vi "Set Shooter RPM.vi"(6 "Key Shot":bool, 8 "Open Loop":bool, 9 "Increment":bool, 10 "Decrement":bool, 11 "Shooter Enabled":bool) -> ()   [LabVIEW 2011]
uses:
  System Set Points and States.vi
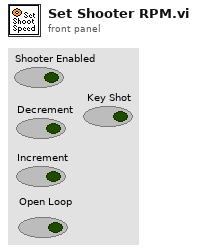
[diagram p1: front panel]
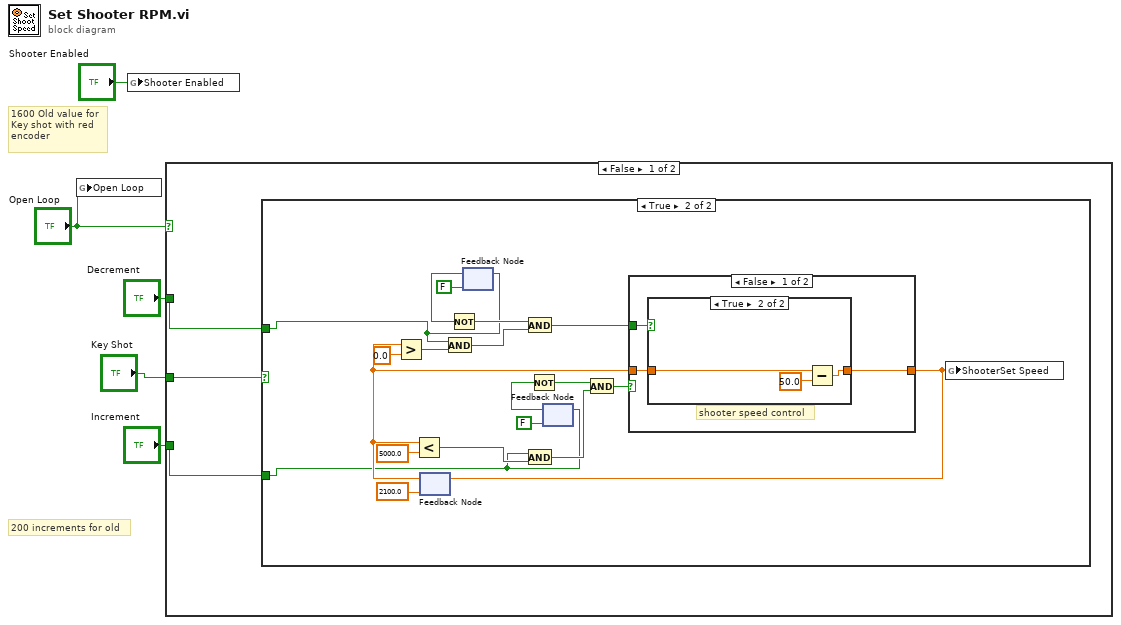
[diagram p0: block diagram]
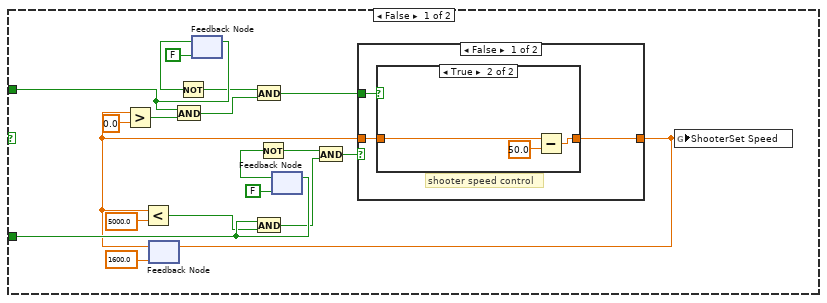
[diagram p2: hidden frame]
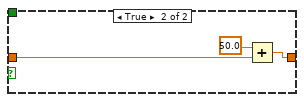
[diagram p4: hidden frame]
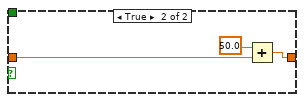
[diagram p6: hidden frame]
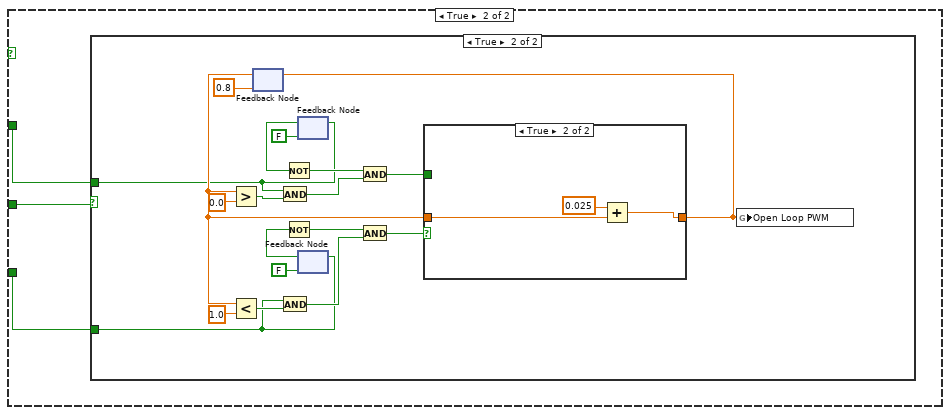
[diagram p7: hidden frame]
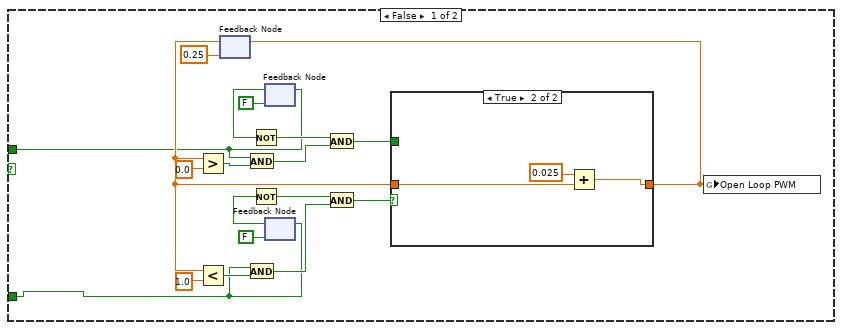
[diagram p8: hidden frame]
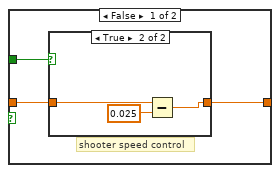
[diagram p9: hidden frame]
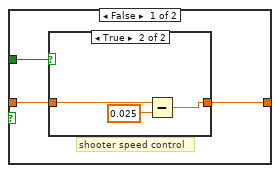
[diagram p11: hidden frame]
diagram:
  # "200 increments for old"
  # "1600 Old value for\nKey shot with red\nencoder"
  n1 = global write "System Set Points and States.vi" "Open Loop"("Open Loop") -> ()
  n2 = global write "System Set Points and States.vi" "Shooter Enabled"("Shooter Enabled") -> ()
  n3 = case shown="False" "Open Loop" {
    tunnel: "Decrement" -> [w8 w69]
    tunnel: "Increment" -> [w7 w68]
    tunnel: "Key Shot" -> [w6 w67]
    frame False {
      n4 = case shown="True" w6 {
        tunnel: w8 -> [w27 w38]
        tunnel: w7 -> [w26 w39]
        frame False {
          n5 = feedback #1(1600.0) -> (w11:dbl)
          n6 = Greater?(x=w11, y=0.0) -> (0:w9:bool)
          n7 = Less?(x=w11, y=5000.0) -> (x < y?=w12:bool)
          n8 = And(x=w27, y=w9) -> (x .and. y?=w18:bool)
          n9 = feedback #2(FALSE) -> (w22:bool)
          n10 = Not(x=w22) -> (.not. x?=w23:bool)
          n11 = feedback-in #2(w27) -> ()
          n12 = And(x=w23, y=w18) -> (x .and. y?=w19:bool)
          n13 = And(x=w26, y=w12) -> (x .and. y?=w15:bool)
          n14 = feedback #3(FALSE) -> (w20:bool)
          n15 = Not(x=w20) -> (.not. x?=w21:bool)
          n16 = feedback-in #3(w26) -> ()
          n17 = And(x=w21, y=w15) -> (x .and. y?=w16:bool)
          n18 = case shown="False" w16 {
            tunnel: w19 -> [w30 _]
            tunnel: w11 -> [w29 w37]
            tunnel: [w28 w35] -> w25
            frame False {
              # "shooter speed control"
              n19 = case shown="True" w30 {
                tunnel: w29 -> [w31 w34]
                tunnel: [w31 w32] -> w28
                frame False {
                }
                frame True {
                  n20 = Subtract(x=w34, y=50.0) -> (x-y=w32:dbl)
                }
              }
            }
            frame True {
              n21 = Add(x=50.0, y=w37) -> (x+y=w35:dbl)
            }
          }
          n22 = feedback-in #1(w25) -> ()
          n23 = global write "System Set Points and States.vi" "ShooterSet Speed"(w25) -> ()
        }
        frame True {
          n24 = feedback #4(2100.0) -> (w42:dbl)
          n25 = Greater?(x=w42, y=0.0) -> (0:w40:bool)
          n26 = Less?(x=w42, y=5000.0) -> (x < y?=w43:bool)
          n27 = And(x=w38, y=w40) -> (x .and. y?=w49:bool)
          n28 = feedback #5(FALSE) -> (w53:bool)
          n29 = Not(x=w53) -> (.not. x?=w54:bool)
          n30 = feedback-in #5(w38) -> ()
          n31 = And(x=w54, y=w49) -> (x .and. y?=w50:bool)
          n32 = And(x=w39, y=w43) -> (x .and. y?=w46:bool)
          n33 = feedback #6(FALSE) -> (w51:bool)
          n34 = Not(x=w51) -> (.not. x?=w52:bool)
          n35 = feedback-in #6(w39) -> ()
          n36 = And(x=w52, y=w46) -> (x .and. y?=w47:bool)
          n37 = case shown="False" w47 {
            tunnel: w50 -> [w59 _]
            tunnel: w42 -> [w58 w66]
            tunnel: [w57 w64] -> w56
            frame False {
              # "shooter speed control"
              n38 = case shown="True" w59 {
                tunnel: w58 -> [w60 w63]
                tunnel: [w60 w61] -> w57
                frame False {
                }
                frame True {
                  n39 = Subtract(x=w63, y=50.0) -> (x-y=w61:dbl)
                }
              }
            }
            frame True {
              n40 = Add(x=50.0, y=w66) -> (x+y=w64:dbl)
            }
          }
          n41 = feedback-in #4(w56) -> ()
          n42 = global write "System Set Points and States.vi" "ShooterSet Speed"(w56) -> ()
        }
      }
    }
    frame True {
      n43 = case shown="True" w67 {
        tunnel: w69 -> [w71 w101]
        tunnel: w68 -> [w70 w100]
        frame False {
          n44 = feedback #7(0.25) -> (w75:dbl)
          n45 = Greater?(x=w75, y=0.0) -> (0:w88:bool)
          n46 = Less?(x=w75, y=1.0) -> (x < y?=w86:bool)
          n47 = And(x=w71, y=w88) -> (x .and. y?=w81:bool)
          n48 = And(x=w70, y=w86) -> (x .and. y?=w83:bool)
          n49 = feedback #8(FALSE) -> (w78:bool)
          n50 = Not(x=w78) -> (.not. x?=w77:bool)
          n51 = feedback-in #8(w71) -> ()
          n52 = feedback #9(FALSE) -> (w80:bool)
          n53 = Not(x=w80) -> (.not. x?=w79:bool)
          n54 = feedback-in #9(w70) -> ()
          n55 = And(x=w77, y=w81) -> (x .and. y?=w74:bool)
          n56 = And(x=w79, y=w83) -> (x .and. y?=w73:bool)
          n57 = case shown="True" w73 {
            tunnel: w74 -> [w91 _]
            tunnel: w75 -> [w90 w98]
            tunnel: [w89 w96] -> w72
            frame False {
              # "shooter speed control"
              n58 = case shown="True" w91 {
                tunnel: w90 -> [w92 w95]
                tunnel: [w92 w93] -> w89
                frame False {
                }
                frame True {
                  n59 = Subtract(x=w95, y=0.025) -> (x-y=w93:dbl)
                }
              }
            }
            frame True {
              n60 = Add(x=0.025, y=w98) -> (x+y=w96:dbl)
            }
          }
          n61 = feedback-in #7(w72) -> ()
          n62 = global write "System Set Points and States.vi" "Open Loop PWM"(w72) -> ()
        }
        frame True {
          n63 = feedback #10(0.8) -> (w104:dbl)
          n64 = Greater?(x=w104, y=0.0) -> (0:w117:bool)
          n65 = Less?(x=w104, y=1.0) -> (x < y?=w115:bool)
          n66 = And(x=w101, y=w117) -> (x .and. y?=w110:bool)
          n67 = And(x=w100, y=w115) -> (x .and. y?=w112:bool)
          n68 = feedback #11(FALSE) -> (w107:bool)
          n69 = Not(x=w107) -> (.not. x?=w106:bool)
          n70 = feedback-in #11(w101) -> ()
          n71 = feedback #12(FALSE) -> (w109:bool)
          n72 = Not(x=w109) -> (.not. x?=w108:bool)
          n73 = feedback-in #12(w100) -> ()
          n74 = And(x=w106, y=w110) -> (x .and. y?=w103:bool)
          n75 = And(x=w108, y=w112) -> (x .and. y?=w102:bool)
          n76 = case shown="True" w102 {
            tunnel: w103 -> [w120 _]
            tunnel: w104 -> [w119 w127]
            tunnel: [w118 w125] -> w99
            frame False {
              # "shooter speed control"
              n77 = case shown="True" w120 {
                tunnel: w119 -> [w121 w124]
                tunnel: [w121 w122] -> w118
                frame False {
                }
                frame True {
                  n78 = Subtract(x=w124, y=0.025) -> (x-y=w122:dbl)
                }
              }
            }
            frame True {
              n79 = Add(x=0.025, y=w127) -> (x+y=w125:dbl)
            }
          }
          n80 = feedback-in #10(w99) -> ()
          n81 = global write "System Set Points and States.vi" "Open Loop PWM"(w99) -> ()
        }
      }
    }
  }
